vi "WORKING_VI_LED.vi"() -> ()   [LabVIEW 2017]
uses:
  <vilib>/myRIO/Instrument Drivers/Onboard IO/DIO/typedefs/DIO Reference.ctl
  <vilib>/myRIO/Common/Instrument Driver Framework/Utilities/typedefs/myRIO Generic Hardware Reference.ctl
  <vilib>/myRIO/Common/Instrument Driver Framework/Utilities/typedefs/Hardware Version Enum.ctl
  <vilib>/myRIO/Common/Instrument Driver Framework/Utilities/typedefs/myRIO v1.0 Reference.ctl
  <vilib>/myRIO/Common/Instrument Driver Framework/Utilities/typedefs/Generic FPGA Reference.ctl
  <vilib>/myRIO/Common/Instrument Driver Framework/myRIO v1.0/DIO/typedefs/DIO Channels List.ctl
  <vilib>/myRIO/Common/Instrument Driver Framework/myRIO v1.0/DIO/typedefs/DIO Channels Enum.ctl
  <vilib>/userdefined/High Color/nirio_resource_hc.ctl
  <vilib>/myRIO/Common/Instrument Driver Framework/Utilities/vis/Is FPGA Ref Available.vi
  <vilib>/myRIO/Common/Instrument Driver Framework/myRIO v1.0/DIO/vis/myRIO v1.1 Open DIO.vi
  <vilib>/myRIO/Instrument Drivers/Onboard IO/DIO/vis/Write.vi
  <vilib>/myRIO/Instrument Drivers/Onboard IO/DIO/vis/Read.vi
  <vilib>/myRIO/Common/Instrument Driver Framework/Utilities/vis/Validate Channels.vi
  <vilib>/myRIO/Common/Instrument Driver Framework/myRIO v1.0/DIO/vis/myRIO v1.0 Reserve DIO.vi
  <vilib>/myRIO/Common/Instrument Driver Framework/myRIO v1.0/Resource Manager/vis/myRIO v1.0 Reserve Channel List.vi
  <vilib>/myRIO/Common/Instrument Driver Framework/myRIO v1.0/DIO/vis/myRIO v1.0 Build MUX Configuration DIO.vi
  <vilib>/myRIO/Common/Instrument Driver Framework/myRIO v1.0/Resource Manager/vis/myRIO v1.0 Reserve Channel.vi
  <vilib>/myRIO/Common/Instrument Driver Framework/myRIO v1.0/Resource Manager/vis/myRIO v1.0 Unreserve Channel.vi
  <vilib>/myRIO/Common/Instrument Driver Framework/myRIO v1.0/Resource Manager/vis/myRIO v1.0 Create Configuration List.vi
  <vilib>/myRIO/Common/Instrument Driver Framework/myRIO v1.0/Resource Manager/vis/myRIO v1.0 Build Mutex Name.vi
  LABVIEW2/killswitch.vi
  <vilib>/Utility/VariantDataType/GetNumericInfo.vi
  <vilib>/Utility/error.llb/Error Cluster From Error Code.vi
  <vilib>/myRIO/Common/Instrument Driver Framework/myRIO v1.0/myRIO v1.1 Open.vi
  <vilib>/myRIO/Common/Instrument Driver Framework/Utilities/vis/IO Manager.vi
  <vilib>/myRIO/Common/Instrument Driver Framework/Utilities/vis/Configuration Manager.vi
  <vilib>/myRIO/Common/Instrument Driver Framework/myRIO v1.0/Resource Manager/vis/myRIO v1.0 Configure IO.vi
  <vilib>/myRIO/Common/Instrument Driver Framework/myRIO v1.0/myRIO v1.0 Close.vi
  <vilib>/myRIO/Common/Instrument Driver Framework/myRIO v1.0/DIO/vis/myRIO v1.0 Write DIO.vi
  <vilib>/myRIO/Common/Instrument Driver Framework/myRIO v1.0/DIO/vis/myRIO v1.0 Read DIO.vi
  <vilib>/myRIO/Express VI/Onboard IO/DO/DO Express VI.xnode
  <vilib>/myRIO/Instrument Drivers/Onboard IO/DIO/vis/myRIO DIO Open.xnode
  <vilib>/myRIO/Express VI/Onboard IO/DI/DI Express VI.xnode
  <vilib>/myRIO/Instrument Drivers/Onboard IO/DIO/DIO.lvlib
panel:
  out "A/DIO7 (Pin 25)":bool
  out "A/DIO6 (Pin 23)":bool
  out "A/DIO5 (Pin 21)":bool
  out "A/DIO4 (Pin 19)":bool
  out "A/DIO3 (Pin 17)":bool
  out "A/DIO2 (Pin 15)":bool
  out "A/DIO1 (Pin 13)":bool
  out "Numeric 2":i32
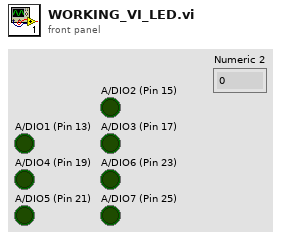
[diagram p1: front panel]
types:
  T1 = typedef "DIO.lvlib/DIO Reference.ctl" = cluster{"myRIO Reference":T2, "DIO Channels List":T6}
  T2 = typedef "myRIO Generic Hardware Reference.ctl" = cluster{"myRIO Model":T3, "myRIO Hardware Reference":T4}
  T3 = typedef "Hardware Version Enum.ctl" = enum16{"Unknown", "myRIO-1900", "myRIO-1950", "roboRIO", "NI ELVIS RIO CM"}
  T4 = typedef "myRIO v1.0 Reference.ctl" = cluster{"Generic FPGA Reference":T5, "Allow multiple opens":bool}
  T5 = typedef "Generic FPGA Reference.ctl" = refnum<k20>
  T6 = typedef "DIO Channels List.ctl" = T7[]
  T7 = typedef "DIO Channels Enum.ctl" = enum16{"Not Connected", "C/DIO0", "C/DIO1", "C/DIO2", "C/DIO3", "C/DIO4", "C/DIO5", "C/DIO6", "C/DIO7", "A/DIO0", "A/DIO1", "A/DIO2", "A/DIO3", "A/DIO4", "A/DIO5", "A/DIO6", "A/DIO7", "A/DIO8", "A/DIO9", "A/DIO10", "A/DIO11", "A/DIO12", "A/DIO13", "A/DIO14", "A/DIO15", "B/DIO0", "B/DIO1", "B/DIO2", "B/DIO3", "B/DIO4", "B/DIO5", "B/DIO6", "B/DIO7", "B/DIO8", "B/DIO9", "B/DIO10", "B/DIO11", "B/DIO12", "B/DIO13", "B/DIO14", "B/DIO15", "LED0", "LED1", "LED2", "LED3", "Button0", "DIO/DIO0", "DIO/DIO1", "DIO/DIO2", "DIO/DIO3", "DIO/DIO4", "DIO/DIO5", "DIO/DIO6", "DIO/DIO7", "DIO/DIO8", "DIO/DIO9", "SPI/CS0", "SPI/CS1", "SPI/CS2", "SPI/CS3", "LED RADIO (Green)", "LED RADIO (Red)", "LED COMM (Green)", "LED COMM (Red)", "LED MODE (Green)", "LED MODE (Red)"}
  T8 = typedef "nirio_resource_hc.ctl" = tag
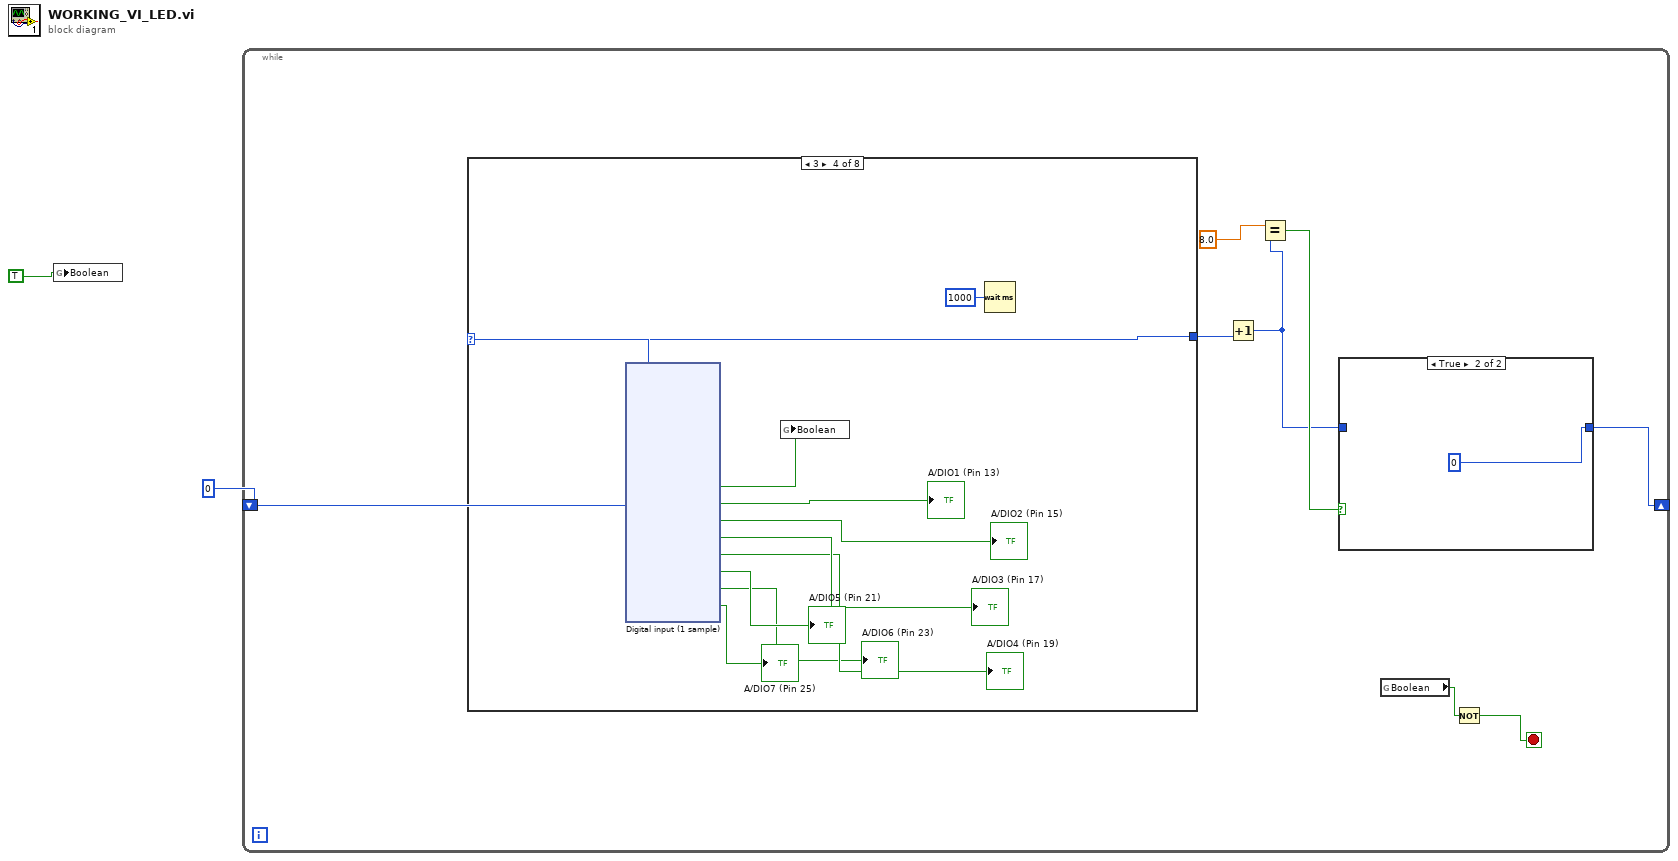
[diagram p0: block diagram]
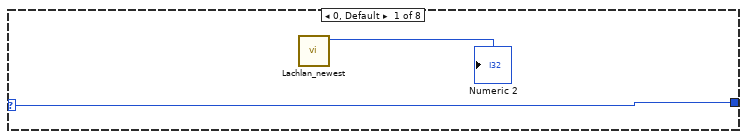
[diagram p3: hidden frame]
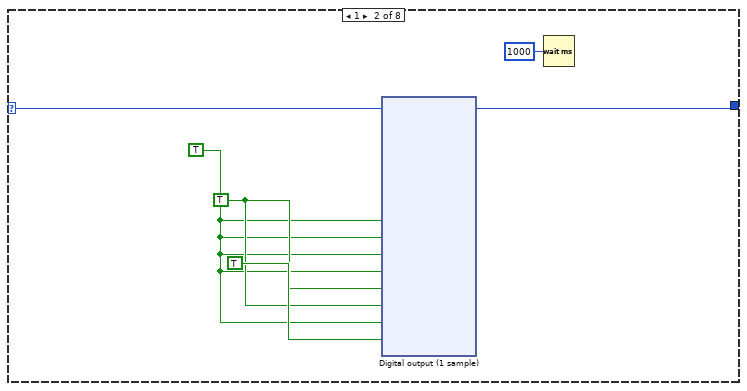
[diagram p4: hidden frame]
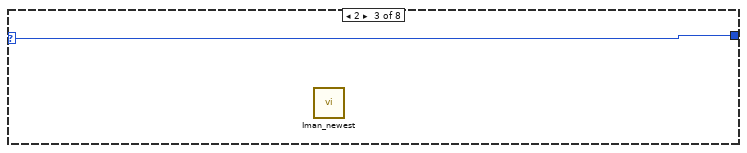
[diagram p5: hidden frame]
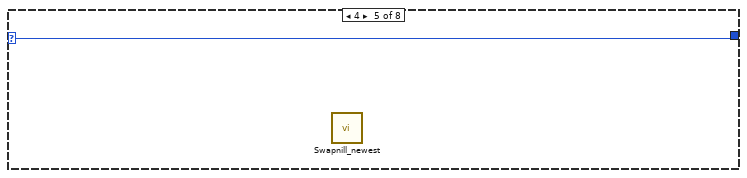
[diagram p6: hidden frame]
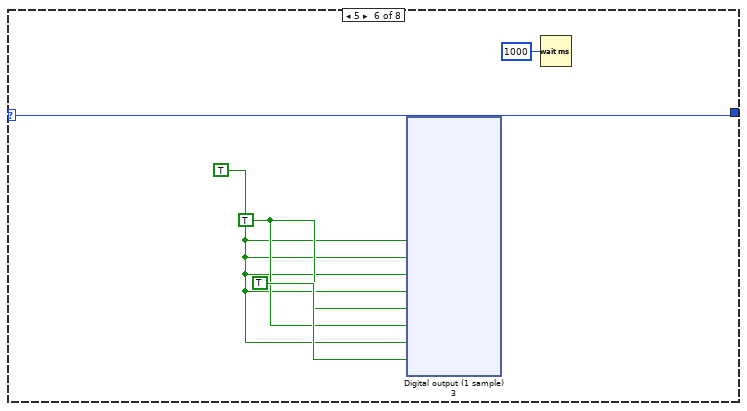
[diagram p7: hidden frame]
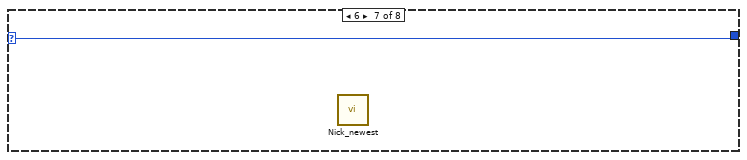
[diagram p8: hidden frame]
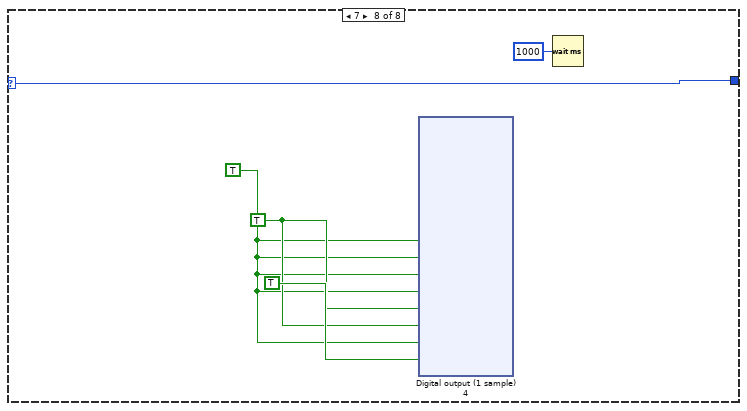
[diagram p9: hidden frame]
diagram:
  n1 = global write "killswitch.vi" "Boolean"(TRUE) -> ()
  n2 = while {
    shift-right: [w5] -> _
    shift-left: 0 -> [w10]
    stop <- w3 stop-if-true
    n3 = case shown="3" w10 {
      selector: w10 -> [w13 w19 w62 w71 w115 w120 w163 w164]
      tunnel: [w13 w19 w62 w71 w115 w120 w163 w164] -> w9
      frame 0, Default {
        n4 = call "Lachlan_newest.vi"() -> ("Numeric"=→"Numeric 2":i32)  [unwired: 11 in]
      }
      frame 1 {
        w16 = TRUE
        w15 = TRUE
        n5 = xnode "Digital output (1 sample)"("A/DIO0 (Pin 11)"=w15, "A/DIO1 (Pin 13)"=w15, "A/DIO2 (Pin 15)"=w15, "A/DIO3 (Pin 17)"=w15, "A/DIO4 (Pin 19)"=w16, "A/DIO5 (Pin 21)"=w16, "A/DIO6 (Pin 23)"=w15, "A/DIO7 (Pin 25)"=TRUE) -> ()  [unwired: 1 in, 1 out]
        n6 = Wait (ms)(milliseconds to wait=u32 1000) -> ()  [unwired: 1 out]
      }
      frame 2 {
        n7 = call "Iman_newest.vi"() -> ()  [unwired: 12 in]
      }
      frame 3 {
        n8 = xnode "Digital input (1 sample)"() -> ("A/DIO0 (Pin 11)"=w63:bool, "A/DIO1 (Pin 13)"=→"A/DIO1 (Pin 13)":bool, "A/DIO2 (Pin 15)"=→"A/DIO2 (Pin 15)":bool, "A/DIO3 (Pin 17)"=→"A/DIO3 (Pin 17)":bool, "A/DIO4 (Pin 19)"=→"A/DIO4 (Pin 19)":bool, "A/DIO5 (Pin 21)"=→"A/DIO5 (Pin 21)":bool, "A/DIO6 (Pin 23)"=→"A/DIO6 (Pin 23)":bool, "A/DIO7 (Pin 25)"=→"A/DIO7 (Pin 25)":bool)  [unwired: 1 in, 1 out]
        n9 = global write "killswitch.vi" "Boolean"(w63) -> ()
        n10 = Wait (ms)(milliseconds to wait=u32 1000) -> ()  [unwired: 1 out]
      }
      frame 4 {
        n11 = call "Swapnill_newest.vi"() -> ()  [unwired: 12 in]
      }
      frame 5 {
        w117 = TRUE
        w116 = TRUE
        n12 = xnode "Digital output (1 sample) 3"("A/DIO0 (Pin 11)"=w116, "A/DIO1 (Pin 13)"=w116, "A/DIO2 (Pin 15)"=w116, "A/DIO3 (Pin 17)"=w116, "A/DIO4 (Pin 19)"=w117, "A/DIO5 (Pin 21)"=w117, "A/DIO6 (Pin 23)"=w116, "A/DIO7 (Pin 25)"=TRUE) -> ()  [unwired: 1 in, 1 out]
        n13 = Wait (ms)(milliseconds to wait=u32 1000) -> ()  [unwired: 1 out]
      }
      frame 6 {
        n14 = call "Nick_newest.vi"() -> ()  [unwired: 12 in]
      }
      frame 7 {
        w166 = TRUE
        w165 = TRUE
        n15 = xnode "Digital output (1 sample) 4"("A/DIO0 (Pin 11)"=w165, "A/DIO1 (Pin 13)"=w165, "A/DIO2 (Pin 15)"=w165, "A/DIO3 (Pin 17)"=w165, "A/DIO4 (Pin 19)"=w166, "A/DIO5 (Pin 21)"=w166, "A/DIO6 (Pin 23)"=w165, "A/DIO7 (Pin 25)"=TRUE) -> ()  [unwired: 1 in, 1 out]
        n16 = Wait (ms)(milliseconds to wait=u32 1000) -> ()  [unwired: 1 out]
      }
    }
    n17 = Increment(x=w9) -> (x+1=w6:i32)
    n18 = Equal?(x=8.0, y=w6) -> (x = y?=w7:bool)
    n19 = case shown="True" w7 {
      tunnel: w6 -> [w11 _]
      tunnel: [w11 0] -> w5
      frame False {
      }
      frame True {
      }
    }
    n20 = global read "killswitch.vi" "Boolean"() -> (w4:bool)
    n21 = Not(x=w4) -> (.not. x?=w3:bool)
  }
